vi "Global 3.vi"() -> ()   [LabVIEW 2012]
panel:
  in  "Array":string[](array[string])
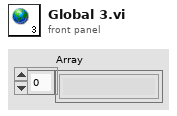
[diagram p1: front panel]
diagram:
